vi "stateManager.vi"() -> ()   [LabVIEW 2020]
uses:
  InstState.ctl
panel:
  out "InstState_IS":T1
  out "last_msg[s]":dbl format="%#_6f"
  in  "outdate[s]":dbl=20.0
  out "msg timestamp\noutdated !":bool
  out "state_n":u16
  out "InstState_SET":T1
  in  "stop":bool
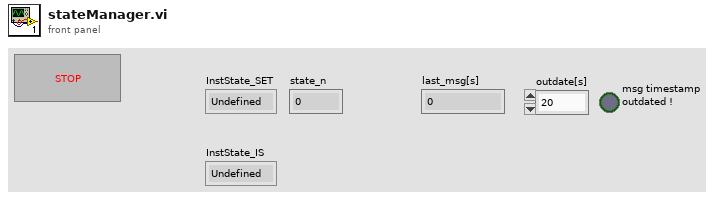
[diagram p1: front panel]
types:
  T1 = typedef "InstState.ctl" = enum16{"Undefined", "Idle", "WarmUp", "Standby", "Measure"}
  T2 = cluster{"sender_IPv4":string, "sender_port":u16, "receiver_IPv4":string, "receiver_port":u16, "msg_len":u16, "timestamp":dbl, "msg_type":u8, "data (bytes string)":string, "cs":u32}
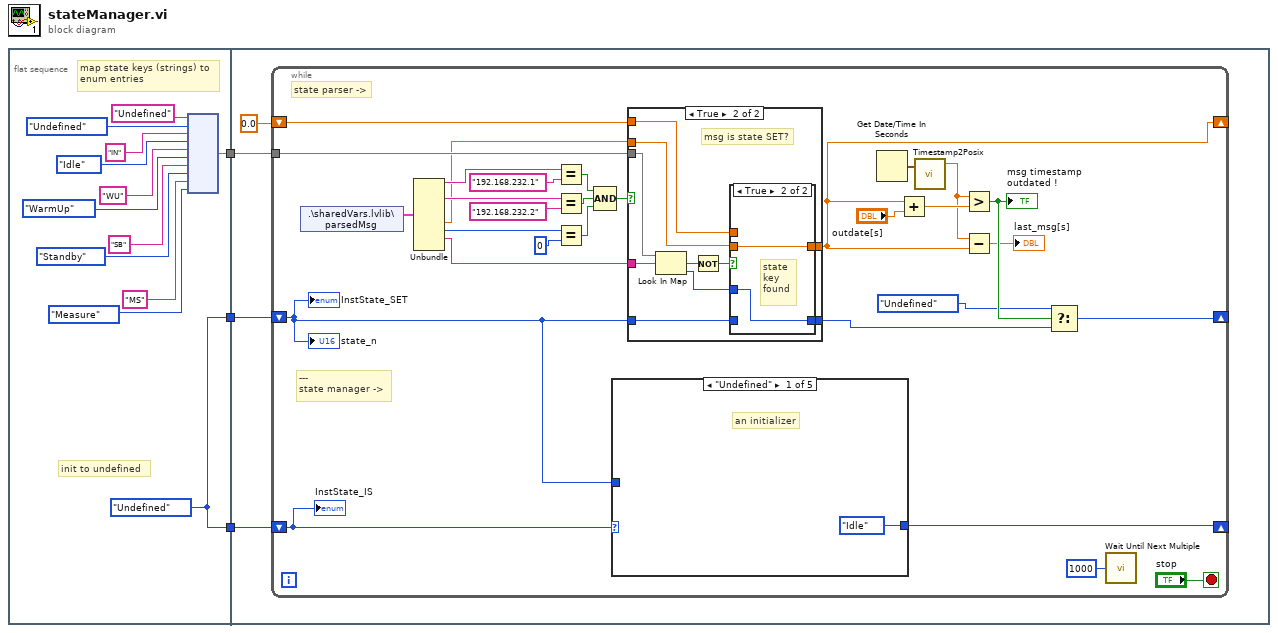
[diagram p0: block diagram]
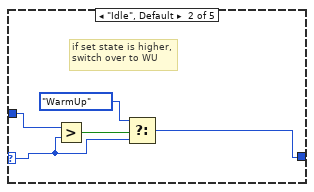
[diagram p2: hidden frame]
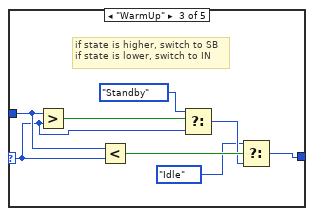
[diagram p3: hidden frame]
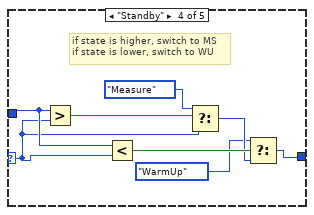
[diagram p4: hidden frame]
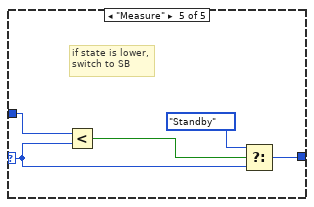
[diagram p5: hidden frame]
diagram:
  n1 = flat-sequence {
    tunnel: [w10] -> w3
    tunnel: [w8] -> w2
    tunnel: [w8] -> w1
    tunnel: w3 -> [w19]
    tunnel: w2 -> [w18]
    tunnel: w1 -> [w17]
    frame #0 {
      w8 = InstState."Undefined" ("InstState")
      # "init to undefined"
      # "map state keys (strings) to\nenum entries"
      n2 = node("Undefined" ("key"), InstState."Undefined" ("InstState"), "IN" ("key"), InstState."Idle" ("InstState"), "WU" ("key"), InstState."WarmUp" ("InstState"), "SB" ("key"), InstState."Standby" ("InstState"), "MS" ("key"), InstState."Measure" ("InstState")) -> (w10:map{string, T1})
    }
    frame #1 {
      n3 = while {
        tunnel: w19 -> [w35]
        shift-right: [w29] -> _
        shift-left: w18 -> [w23]
        shift-right: [w24] -> _
        shift-left: w17 -> [w25]
        shift-right: [w20] -> _
        shift-left: 0.0 ("timestamp") -> [w21]
        stop <- "stop" stop-if-true
        # "---\nstate manager ->"
        # "state parser ->"
        n4 = shared-variable ".\\sharedVars.lvlib\\parsedMsg"() -> (w47:T2)  [unwired: 1 in, 1 out]
        n5 = Unbundle(w47) -> ("sender_IPv4"=w44:string, "receiver_IPv4"=w42:string, "timestamp"=w22:dbl, "msg_type"=w46:u8, "data (bytes string)"=w36:string)  [unwired: 4 out]
        n6 = Equal?(x=w44, y="192.168.232.1") -> (x = y?=w40:bool)
        n7 = Equal?(x=w42, y="192.168.232.2") -> (x = y?=w39:bool)
        n8 = Equal?(x=w46, y=u8 0) -> (x = y?=w38:bool)
        n9 = Compound Arithmetic op=AND(w40, w39, w38) -> (w37:bool)
        n10 = case shown="\"Undefined\"" w25 {
          selector: w25 -> [_ w53 w59 w64 w73]
          tunnel: [InstState."Idle" ("InstState") w51 w56 w66 w75] -> w24
          tunnel: w23 -> [_ w55 w61 w65 w76]
          frame "Undefined" {
            # "an initializer"
          }
          frame "Idle", Default {
            # "if set state is higher,\nswitch over to WU"
            n11 = Greater?(x=w55, y=w53) -> (0:w54:bool)
            n12 = Select(t=InstState."WarmUp" ("InstState"), s=w54, f=w53) -> (s? t:f=w51:T1)
          }
          frame "WarmUp" {
            # "if state is higher, switch to SB\nif state is lower, switch to IN"
            n13 = Greater?(x=w61, y=w59) -> (0:w63:bool)
            n14 = Less?(x=w61, y=w59) -> (x < y?=w60:bool)
            n15 = Select(t=InstState."Standby" ("InstState"), s=w63, f=w59) -> (s? t:f=w58:T1)
            n16 = Select(t=InstState."Idle", s=w60, f=w58) -> (s? t:f=w56:T1)
          }
          frame "Standby" {
            # "if state is higher, switch to MS\nif state is lower, switch to WU"
            n17 = Greater?(x=w65, y=w64) -> (0:w71:bool)
            n18 = Less?(x=w65, y=w64) -> (x < y?=w69:bool)
            n19 = Select(t=InstState."Measure" ("InstState"), s=w71, f=w64) -> (s? t:f=w68:T1)
            n20 = Select(t=InstState."WarmUp", s=w69, f=w68) -> (s? t:f=w66:T1)
          }
          frame "Measure" {
            # "if state is lower,\nswitch to SB"
            n21 = Less?(x=w76, y=w73) -> (x < y?=w74:bool)
            n22 = Select(t=InstState."Standby", s=w74, f=w73) -> (s? t:f=w75:T1)
          }
        }
        n23 = case shown="True" w37 {
          tunnel: w36 -> [_ w88]
          tunnel: w35 -> [_ w87]
          tunnel: w23 -> [w78 w83]
          tunnel: [w78 w82] -> w30
          tunnel: w22 -> [_ w81]
          tunnel: w21 -> [w77 w79]
          tunnel: [w77 w80] -> w20
          frame False {
          }
          frame True {
            # "msg is state SET?"
            n24 = Look In Map(map=w87, key=w88) -> (key not found?=w86:bool, value=w84:T1)  [unwired: 1 in]
            n25 = Not(x=w86) -> (.not. x?=w85:bool)
            n26 = case shown="True" w85 {
              tunnel: w84 -> [_ w92]
              tunnel: w83 -> [w90 _]
              tunnel: [w90 w92] -> w82
              tunnel: [w89 w91] -> w80
              tunnel: w81 -> [_ w91]
              tunnel: w79 -> [w89 _]
              frame False {
                # "state\nkey\nnot found!"
              }
              frame True {
                # "state\nkey\nfound"
              }
            }
          }
        }
        n27 = Get Date/Time In Seconds() -> (seconds since 1Jan1904=w34:timestamp)
        n28 = Add(x=w20, y="outdate[s]") -> (x+y=w33:dbl)
        n29 = call "Timestamp2Posix.vi"("timestamp"=w34) -> ("POSIX"=w28:dbl)  [unwired: 4 in]
        n30 = Greater?(x=w28, y=w33) -> (0:w31:bool)
        "msg timestamp\noutdated !" <- w31
        n31 = Subtract(x=w28, y=w20) -> (x-y=→"last_msg[s]":dbl)
        n32 = Select(t=InstState."Undefined" ("InstState"), s=w31, f=w30) -> (s? t:f=w29:T1)
        n33 = call "Wait Until Next Multiple"("Count(mSec)"=u32 1000) -> ()  [unwired: 1 out]
        "InstState_SET" <- w23
        "state_n" <- w23
        "InstState_IS" <- w25
      }
    }
  }
